vi "RSZVB Get Virtual Transform Ground Loop.vi"(6 "Parameter Type (0)":i32(ring) items=["Capacitance", "Inductance", "Resistance"], 7 "Circuit Model (1)":i32(ring)=1 items=["Shunt L"=1, "Shunt C"=2], 8 "error in (no error)":errorcluster {"code" format="%.0x"}, 9 "Function Type (0)":i32(ring) items=["Deembedding", "Embedding"], 10 "Channel (1)":i32=1, 11 "VISA session":refnum<visa-resource-name>) -> (0 "error out":errorcluster {"code" format="%.0x"}, 1 "Ground Loop Value":dbl format="%^.3e", 3 "dup VISA session":refnum<visa-resource-name>)   [LabVIEW 2011]
doc: "This VI returns the capacitance C, inductance L or resistance R value in the different circuit models for ground loop deembedding/embedding.\n\nRemote-control command(s):\nCALCulate<Ch>:TRANsform:VNETworks:GLOop:DEEMbedding:PARameters:C? SC\nCALCulate<Ch>:TRANsform:VNETworks:GLOop:DEEMbedding:PARameters:L? SL\nCALCulate<Ch>:TRANsform:VNETworks:GLOop:DEEMbedding:PARameters:R? SC | SL\nCALCulate<Ch>:TRANsform:VNETworks:GLOop:EMBedding:PARameters:C? SC\nCALCulate<Ch>:TRANsform:VNETworks:GLOop:EMBedding:PARameters:L? SL\nCALCulate<Ch>:TRANsform:VNETworks:GLOop:EMBedding:PARameters:R? SC | SL"
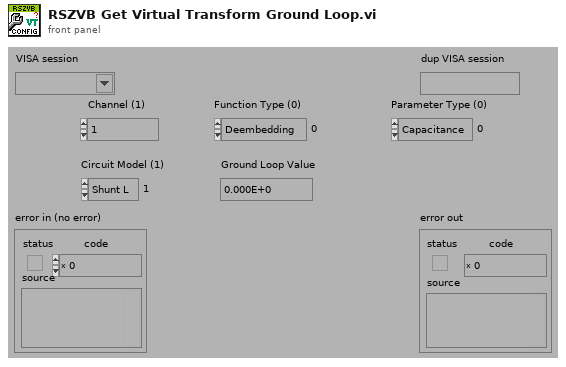
[diagram p1: front panel]
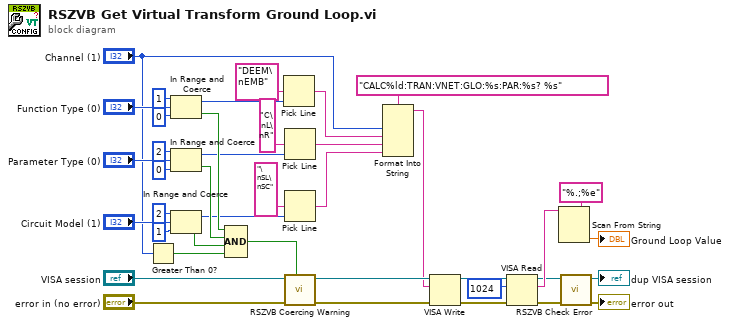
[diagram p0: block diagram]
diagram:
  n1 = Greater Than 0?(x="Channel (1)") -> (x > 0?=w15:bool)
  n2 = In Range and Coerce(upper limit=1, x="Function Type (0)", lower limit=0) -> (coerced(x)=w30:i32, In Range?=w26:bool)
  n3 = In Range and Coerce(upper limit=2, x="Parameter Type (0)", lower limit=0) -> (coerced(x)=w17:i32, In Range?=w27:bool)
  n4 = In Range and Coerce(upper limit=2, x="Circuit Model (1)", lower limit=1) -> (coerced(x)=w22:i32, In Range?=w28:bool)
  n5 = Compound Arithmetic op=AND(w26, w27, w28, w15) -> (w11:bool)
  n6 = Pick Line(multi-line string="DEEM\nEMB", line index=w30) -> (output string=w25:string)  [unwired: 1 in]
  n7 = Pick Line(multi-line string="C\nL\nR", line index=w17) -> (output string=w24:string)  [unwired: 1 in]
  n8 = Pick Line(multi-line string="\nSL\nSC", line index=w22) -> (output string=w21:string)  [unwired: 1 in]
  n9 = call "RSZVB Coercing Warning.vi"("In Range?"=w11, "error in (no error)"="error in (no error)", "VISA session"="VISA session") -> ("error out"=w38:errorcluster, "dup VISA session"=w39:refnum<visa-resource-name>)  [unwired: 7 in]
  n10 = Format Into String(format string="CALC%ld:TRAN:VNET:GLO:%s:PAR:%s? %s", "Channel (1)", w25, w24, w21) -> (resulting string=w20:string)  [unwired: 2 in, 1 out]
  n11 = VISA Write(VISA resource name=w39, write buffer=w20, error in (no error)=w38) -> (VISA resource name out=w4:refnum<visa-resource-name>, error out=w5:errorcluster)  [unwired: 1 out]
  n12 = VISA Read(VISA resource name=w4, byte count=u32 1024 ("byte count (0)"), error in (no error)=w5) -> (VISA resource name out=w7:refnum<visa-resource-name>, read buffer=w10:string, error out=w8:errorcluster)  [unwired: 1 out]
  n13 = Scan From String(format string="%.;%e", input string=w10) -> (output 1=→"Ground Loop Value":dbl)  [unwired: 3 in, 3 out]
  n14 = call "RSZVB Check Error.vi"("error in (no error)"=w8, "VISA session"=w7) -> ("error out"=→"error out":errorcluster, "dup VISA session"=→"dup VISA session":refnum<visa-resource-name>)  [unwired: 8 in]
